vi "MR_analysis_interpol_solver_dataview.vi"(5 "Raw data Y(X) at different Z":cluster{"all rows":dbl[], "all rows":dbl[]}[](graph)) -> ()   [LabVIEW 2025]
panel:
  in  "factor":i32=11
  in  "method":T1(ring)
  in  "Uniform X":bool
  in  "X table":string
  in  "step X":sgl=3.0 format="%.3f"
  in  "final X":sgl=7.0 format="%.2f"
  in  "stop":bool
  in  "Enum":T2(ring)
  out "Y(Z) at different X":cluster{"all rows":dbl[], "all rows":dbl[]}[](graph)=[{"all rows"=[4.2, 3.5, 3.0, 2.5, 2.2, 1.9, 1.7, 1.5, 1.37, 1.2, 1.1, 1.0, 0.9, 0.8, 0.7, 0.6, 0.48], "all rows"=[inf, inf, inf, inf, inf, inf, inf, inf, inf, inf, inf, inf, inf, inf, inf, inf, inf]}, {"all rows"=[4.2, 3.5, 3.0, 2.5, 2.2, 1.9, 1.7, 1.5, 1.37, 1.2, 1.1, 1.0, 0.9, 0.8, 0.7, 0.6, 0.48], "all rows"=[inf, inf, inf, inf, inf, inf, inf, inf, inf, inf, inf, inf, inf, inf, inf, inf, inf]}, {"all rows"=[4.2, 3.5, 3.0, 2.5, 2.2, 1.9, 1.7, 1.5, 1.37, 1.2, 1.1, 1.0, 0.9, 0.8, 0.7, 0.6, 0.48], "all rows"=[inf, inf, inf, inf, inf, inf, inf, inf, inf, inf, inf, inf, inf, inf, inf, inf, inf]}]
  in  "initial X":sgl=0.01 format="%.2f"
  in  "z parameters\n(needed)":string="0\n0.48\n0.96\n1.92\n3.84\n4.08\n4.08\n4.32\n4.56\n4.8\n5.04\n5.28\n5.52\n5.76\n6\n6.24\n6.48\n6.72\n6.96\n7.44\n8.16\n9.12\n10.56\n12.48\n14.4\n18.24\n23.04\n27.84\n32.64\n37.44\n42.24\n47.04\n51.84\n56.64\n61.44\n66.24\n75.84\n85.44\n95.04"
  # "X-table"
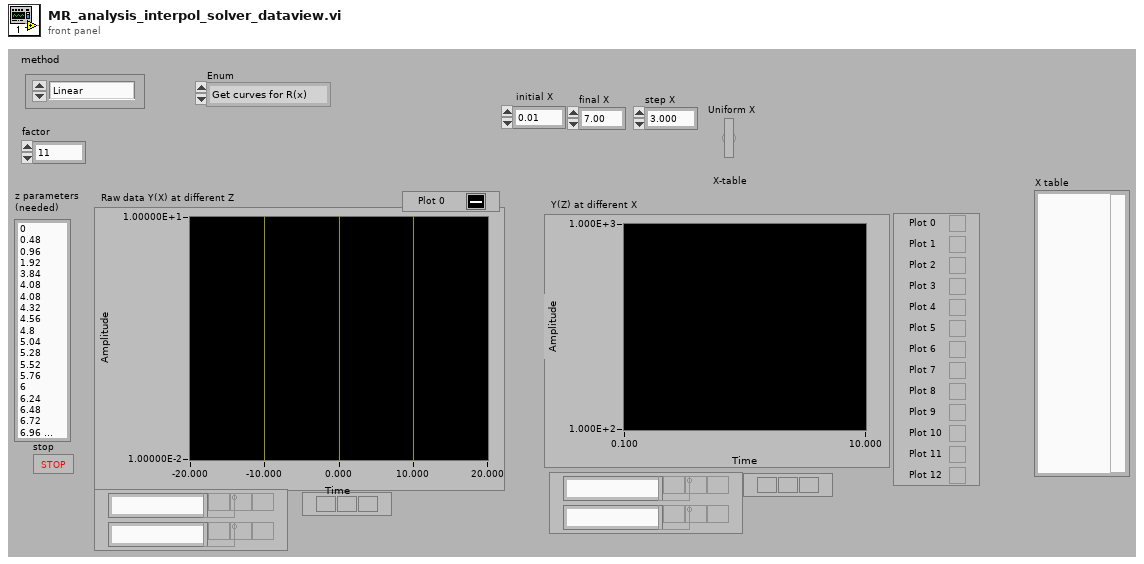
[diagram p1: front panel]
types:
  T1 = enum16{"Linear", "Polynomial", "Spline", "Rational"}
  T2 = enum16{"Get curves for R(x)", "extremum in deriv"}
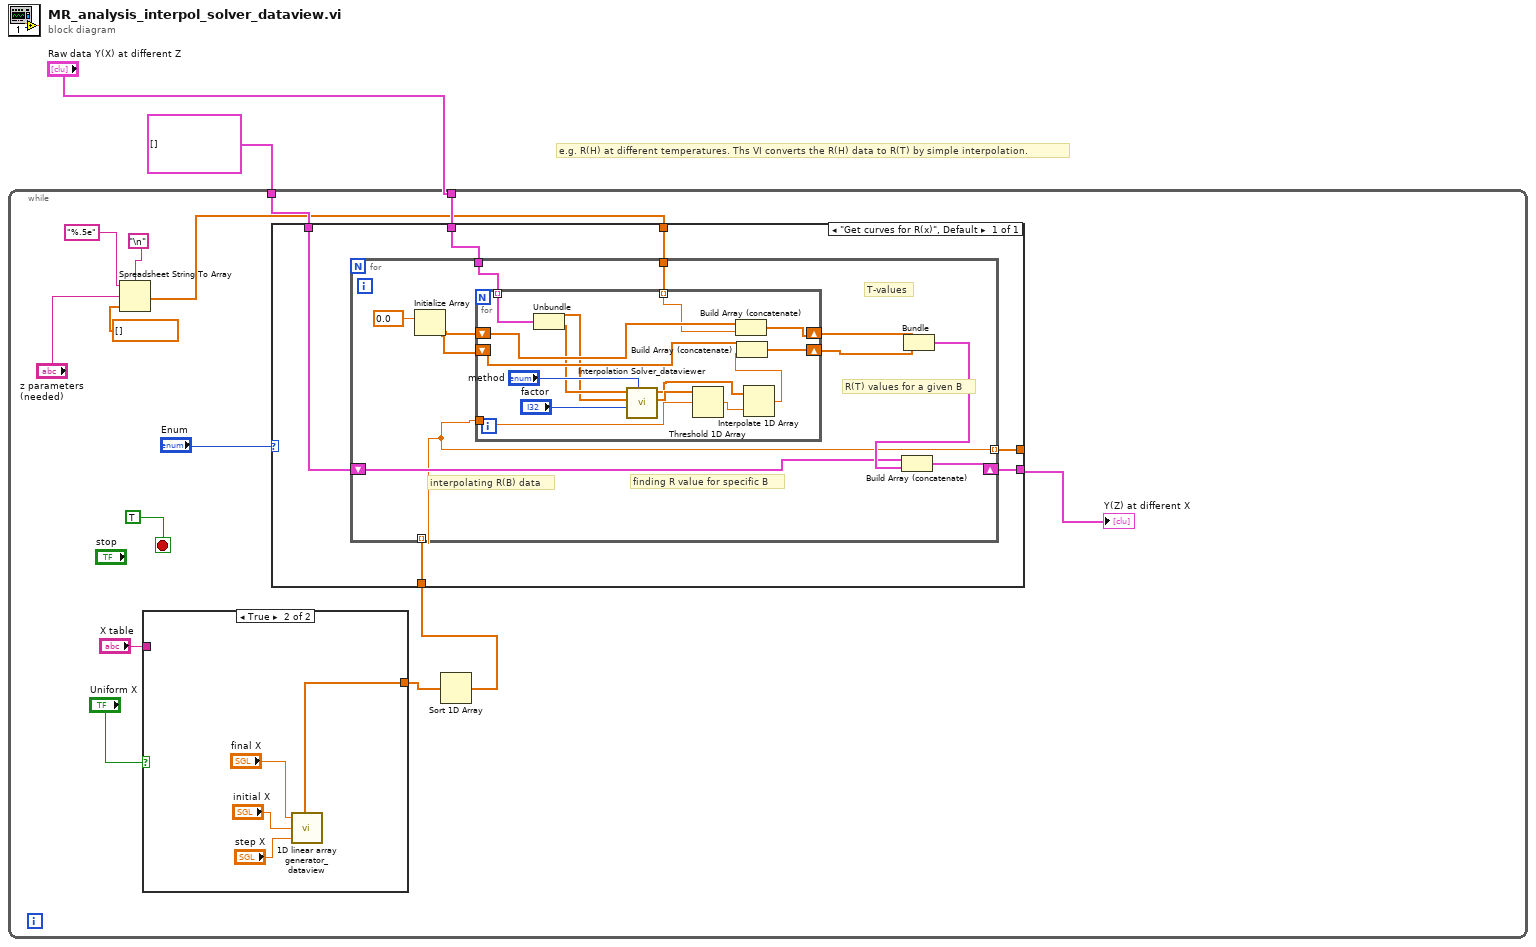
[diagram p0: block diagram]
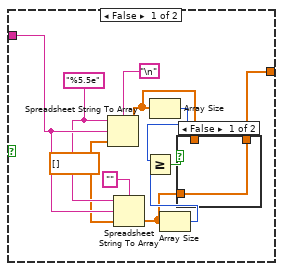
[diagram p2: hidden frame]
diagram:
  # "e.g. R(H) at different temperatures. Ths VI converts the R(H) data to R(T) by simple interpolation."
  n1 = while {
    tunnel: "Raw data Y(X) at different Z" -> [w15]
    tunnel: cluster{"all rows":sgl[], "all rows":sgl[]}[] [] -> [w14]
    stop <- TRUE stop-if-true
    n2 = Spreadsheet String To Array(delimiter (Tab)="\n", format string="%.5e", spreadsheet string="z parameters\n(needed)", array type (2D Dbl)=dbl[] []) -> (array=w6:dbl[])
    n3 = case shown="True" "Uniform X" {
      tunnel: [w18 w30] -> w11
      tunnel: "X table" -> [w26 _]
      frame False {
        w24 = dbl[] []
        w25 = "%5.5e" ("format string")
        n4 = Spreadsheet String To Array(delimiter (Tab)="\n", format string=w25, spreadsheet string=w26, array type (2D Dbl)=w24) -> (array=w19:dbl[])
        n5 = Spreadsheet String To Array(delimiter (Tab)="", format string=w25, spreadsheet string=w26, array type (2D Dbl)=w24) -> (array=w17:dbl[])
        n6 = Array Size(array=w19) -> (size(s)=w22:i32)
        n7 = Array Size(array=w17) -> (size(s)=w21:i32)
        n8 = Greater Or Equal?(x=w22, y=w21) -> (x >= y?=w20:bool)
        n9 = case shown="False" w20 {
          tunnel: w19 -> [_ w29]
          tunnel: [w28 w29] -> w18
          tunnel: w17 -> [w28 _]
          frame False {
          }
          frame True {
          }
        }
      }
      frame True {
        n10 = call "1D linear array generator_dataview.vi"("step X"="step X", "initial X"="initial X", "final X"="final X") -> ("Array"=w30:dbl[])
      }
    }
    n11 = Sort 1D Array(array=w11) -> (sorted array=w10:dbl[])
    n12 = case shown="\"Get curves for R(x)\", Default" "Enum" {
      tunnel: w15 -> [w37]
      tunnel: w14 -> [w35]
      tunnel: [w39] -> w13
      tunnel: w6 -> [w38]
      tunnel: [w36] -> _
      tunnel: w10 -> [w34]
      frame "Get curves for R(x)", Default {
        n13 = for {
          tunnel: w37 -> [w49]
          shift-right: [w45] -> w39
          shift-left: w35 -> [w44]
          tunnel: w38 -> [w43]
          tunnel: [w41] -> w36 mode=indexing
          tunnel: w34 -> [w41] mode=indexing
          # "T-values"
          # "R(T) values for a given B"
          # "finding R value for specific B"
          # "interpolating R(B) data"
          n14 = Initialize Array(0.0 ("element")) -> (w47:dbl[])  [unwired: 1 in]
          n15 = for {
            tunnel: w49 -> [w64] mode=indexing
            shift-right: [w60] -> w40
            shift-left: w47 -> [w61]
            tunnel: w41 -> [w53]
            shift-right: [w62] -> w42
            shift-left: w47 -> [w63]
            tunnel: w43 -> [w59] mode=indexing
            n16 = Unbundle(w64) -> ("all rows"=w55:dbl[], "all rows"=w56:dbl[])
            n17 = call "Interpolation Solver_dataviewer.vi"("method"="method", "factor"="factor", "x-original"=w55, "y-original"=w56) -> ("x-interpolated"=w54:dbl[], "y-interpolated"=w52:dbl[])  [unwired: 6 in]
            n18 = Threshold 1D Array(2:w53, 3:w54) -> (0:w51:dbl)  [unwired: 1 in]
            n19 = Build Array (concatenate)(w61, w59) -> (w60:dbl[])
            n20 = Interpolate 1D Array(1:w51, 2:w52) -> (0:w50:dbl)
            n21 = Build Array (concatenate)(w63, w50) -> (w62:dbl[])
          }
          n22 = Bundle(w40, w42) -> (w46:cluster{dbl[], dbl[]})  [unwired: 1 in]
          n23 = Build Array (concatenate)(w44, w46) -> (w45:cluster{"all rows":dbl[], "all rows":dbl[]}[])
        }
      }
    }
    "Y(Z) at different X" <- w13
  }
